vi "02_main.vi"() -> ()   [LabVIEW 2011]
panel:
  in  "Array":i32[](array[numeric])
  out "Enum":enum16{"run", "stop", "init", "error"}(ring)
  in  "running":bool
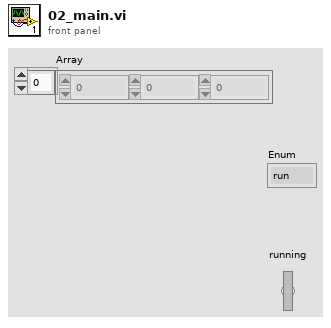
[diagram p1: front panel]
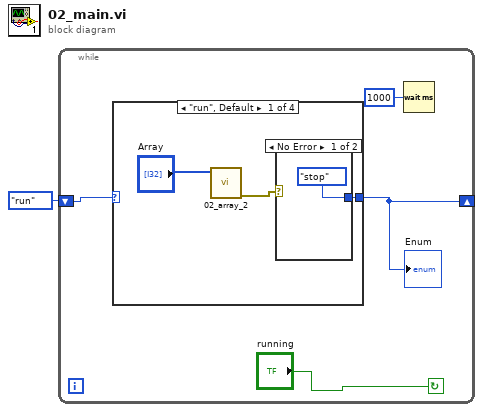
[diagram p0: block diagram]
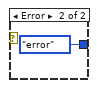
[diagram p2: hidden frame]
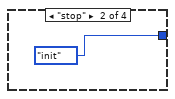
[diagram p3: hidden frame]
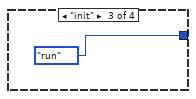
[diagram p4: hidden frame]
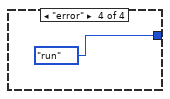
[diagram p5: hidden frame]
diagram:
  n1 = while {
    shift-right: [w2] -> _
    shift-left: enum16{"run", "stop", "init", "error"}."run" -> [w3]
    stop <- "running" continue-if-true
    n2 = case shown="\"run\", Default" w3 {
      tunnel: [w8 enum16{"run", "stop", "init", "error"}."init" enum16{"run", "stop", "init", "error"}."run" enum16{"run", "stop", "init", "error"}."run"] -> w2
      frame "run", Default {
        n3 = call "02_array_2.vi"("ArrayIn"="Array") -> ("errorOut"=w6:errorcluster)  [unwired: 9 in, 1 out]
        n4 = case shown="No Error" w6 {
          tunnel: [enum16{"run", "stop", "init", "error"}."stop" enum16{"run", "stop", "init", "error"}."error"] -> w8
          frame No Error {
          }
          frame Error {
          }
        }
      }
      frame "stop" {
      }
      frame "init" {
      }
      frame "error" {
      }
    }
    "Enum" <- w2
    n5 = Wait (ms)(milliseconds to wait=u32 1000) -> ()  [unwired: 1 out]
  }
